vi "filter seq channels by readers.vi"(9 "include? (default: exclude)":bool, 10 "readers":string[](array[string]), 11 "engine configuration in":refnum<class "base TBM sequencer configuration.lvclass">) -> (2 "seq channels":refnum<class "TBM channel.lvclass">[](array[class]), 3 "engine configuration out":refnum<class "base TBM sequencer configuration.lvclass">)   [LabVIEW 2014, in "base TBM sequencer configuration.lvclass"]
uses:
  base TBM sequencer configuration.lvclass
  <vilib>/NI/Tag Bus Module Framework/channel/TBM channel.lvclass
  base TBM sequencer configuration.lvclass/base TBM sequencer configuration.ctl
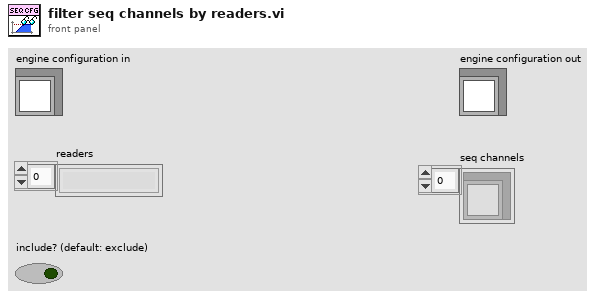
[diagram p1: front panel]
types:
  T1 = typedef "base TBM sequencer configuration.lvclass/Tag Info.ctl" = cluster{"Channel":refnum<class "TBM channel.lvclass">, "Writers":string[], "Readers":string[], "Owning ID":string}
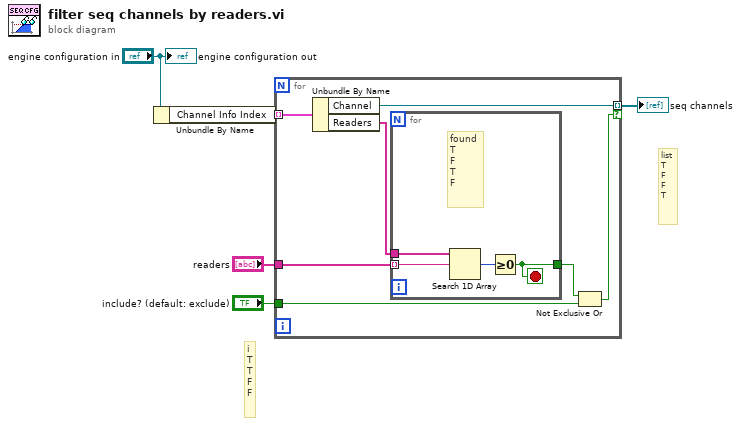
[diagram p0: block diagram]
diagram:
  # "list\nT\nF\nF\nT"
  # "i\nT\nT\nF\nF"
  n1 = Unbundle By Name("engine configuration in") -> ("Channel Info Index"=w4:T1[])
  n2 = for {
    tunnel: w4 -> [w12] mode=indexing
    tunnel: [w11] -> w3 mode=indexing if=w6
    tunnel: "readers" -> [w10]
    tunnel: "include? (default: exclude)" -> [w7]
    n3 = Unbundle By Name(w12) -> ("Channel"=w11:refnum<class "TBM channel.lvclass">, "Readers"=w9:string[])
    n4 = for {
      tunnel: w10 -> [w15] mode=indexing
      tunnel: w9 -> [w14]
      tunnel: [w13] -> w8
      stop <- w13 stop-if-true
      # "found\nT\nF\nT\nF"
      n5 = Search 1D Array(1D array=w14, element=w15) -> (index of element=w16:i32)  [unwired: 1 in]
      n6 = Greater Or Equal To 0?(x=w16) -> (x >= 0?=w13:bool)
    }
    n7 = Not Exclusive Or(1:w7, 2:w8) -> (0:w6:bool)
  }
  "seq channels" <- w3
  "engine configuration out" <- "engine configuration in"
